vi "pH电极校准.vi"() -> ()   [LabVIEW 2016, in "国弘多参数.lvlib"]
uses:
  <vilib>/Analysis/NI_AALBase.lvlib
panel:
  out "变异系数":dbl
  out "standard deviation":dbl caption="标准差" format="%0.2f"
  out "mean":dbl caption="均值" format="%0.2f"
  out "当前检测值":dbl
  out "提示":string
  in  "第二点通过校正":bool
  in  "第一点通过校正":bool
  in  "第二点校正":bool
  in  "第一点校正":bool
  out "标液2":dbl
  out "标液1":dbl
  out "当前信号值":dbl
  out "偏移值补偿":dbl
  out "电极斜率":dbl
  out "电极零点":dbl
  # "酸碱度电极设定"
  # "mV"
  # "pH"
  # "%"
  # "mV"
  # "电极校正"
  # "标准液值:"
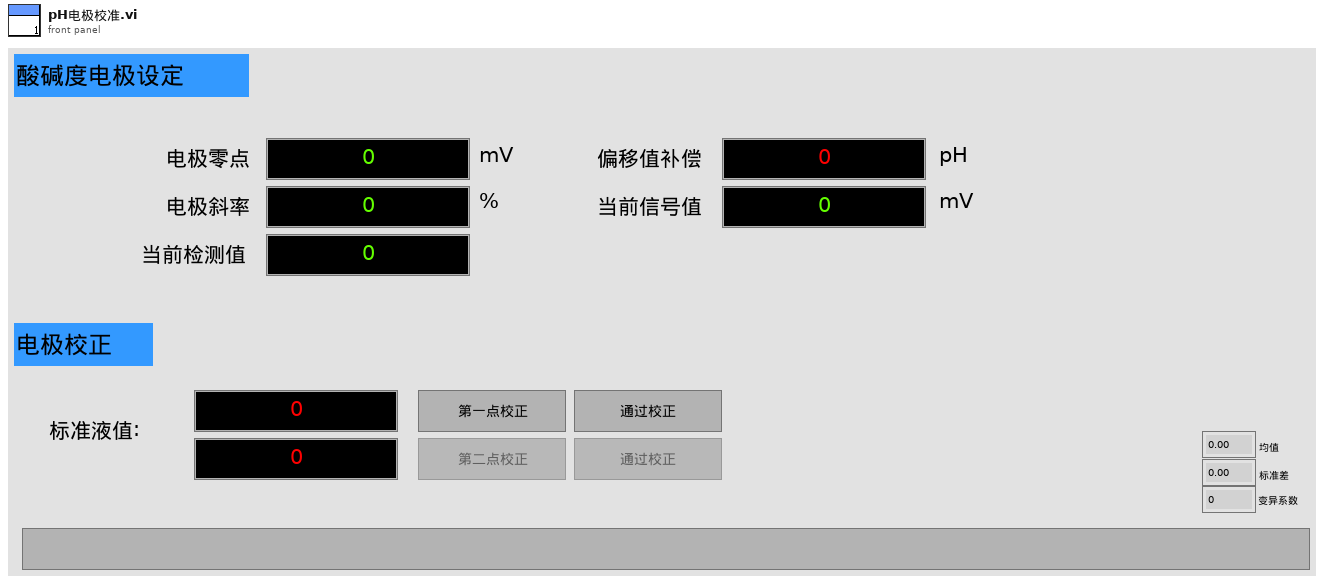
[diagram p1: front panel]
types:
  T1 = typedef "国弘多参数.lvlib/校准步骤.ctl" = enum16{"待机", "第一点校准启动", "第二点校准启动", "第一点校准写入", "第二点校准写入", "第一点校准失败", "第二点校准失败"}
  T2 = enum8{"Enabled", "Disabled", "Disabled and Grayed Out"}
  T3 = cluster{"电极状态标志":u16, "电极型号标志":u16, "酸碱度测量值":sgl, "温度测量值":sgl, "酸碱度信号值":sgl, "温度信号值":sgl, "酸碱度偏移修正值":sgl, "温度偏移修正值":sgl, "手动温度补偿值":sgl, "酸碱度电极零点":sgl, "酸碱度电极斜率":sgl, "第1点标准值记录":sgl, "第1点信号值记录":sgl, "第1点温度值记录":sgl, "第2点标准值记录":sgl, "第2点信号值记录":sgl, "第2点温度值记录":sgl, "命令滤波设定":u16, "温度模式":enum16{"ATC", "MTC"}, "生产批次":u16, "电极序号":u16, "串口地址":u16, "串口波特率":enum16{"9600", "19200", "115200"}, "串口校验位":enum16{"NONE", "ODD", "EVEN"}, "串口停止位":enum16{"1bit", "2bit"}, "第一点标准值":sgl, "第二点标准值":sgl}
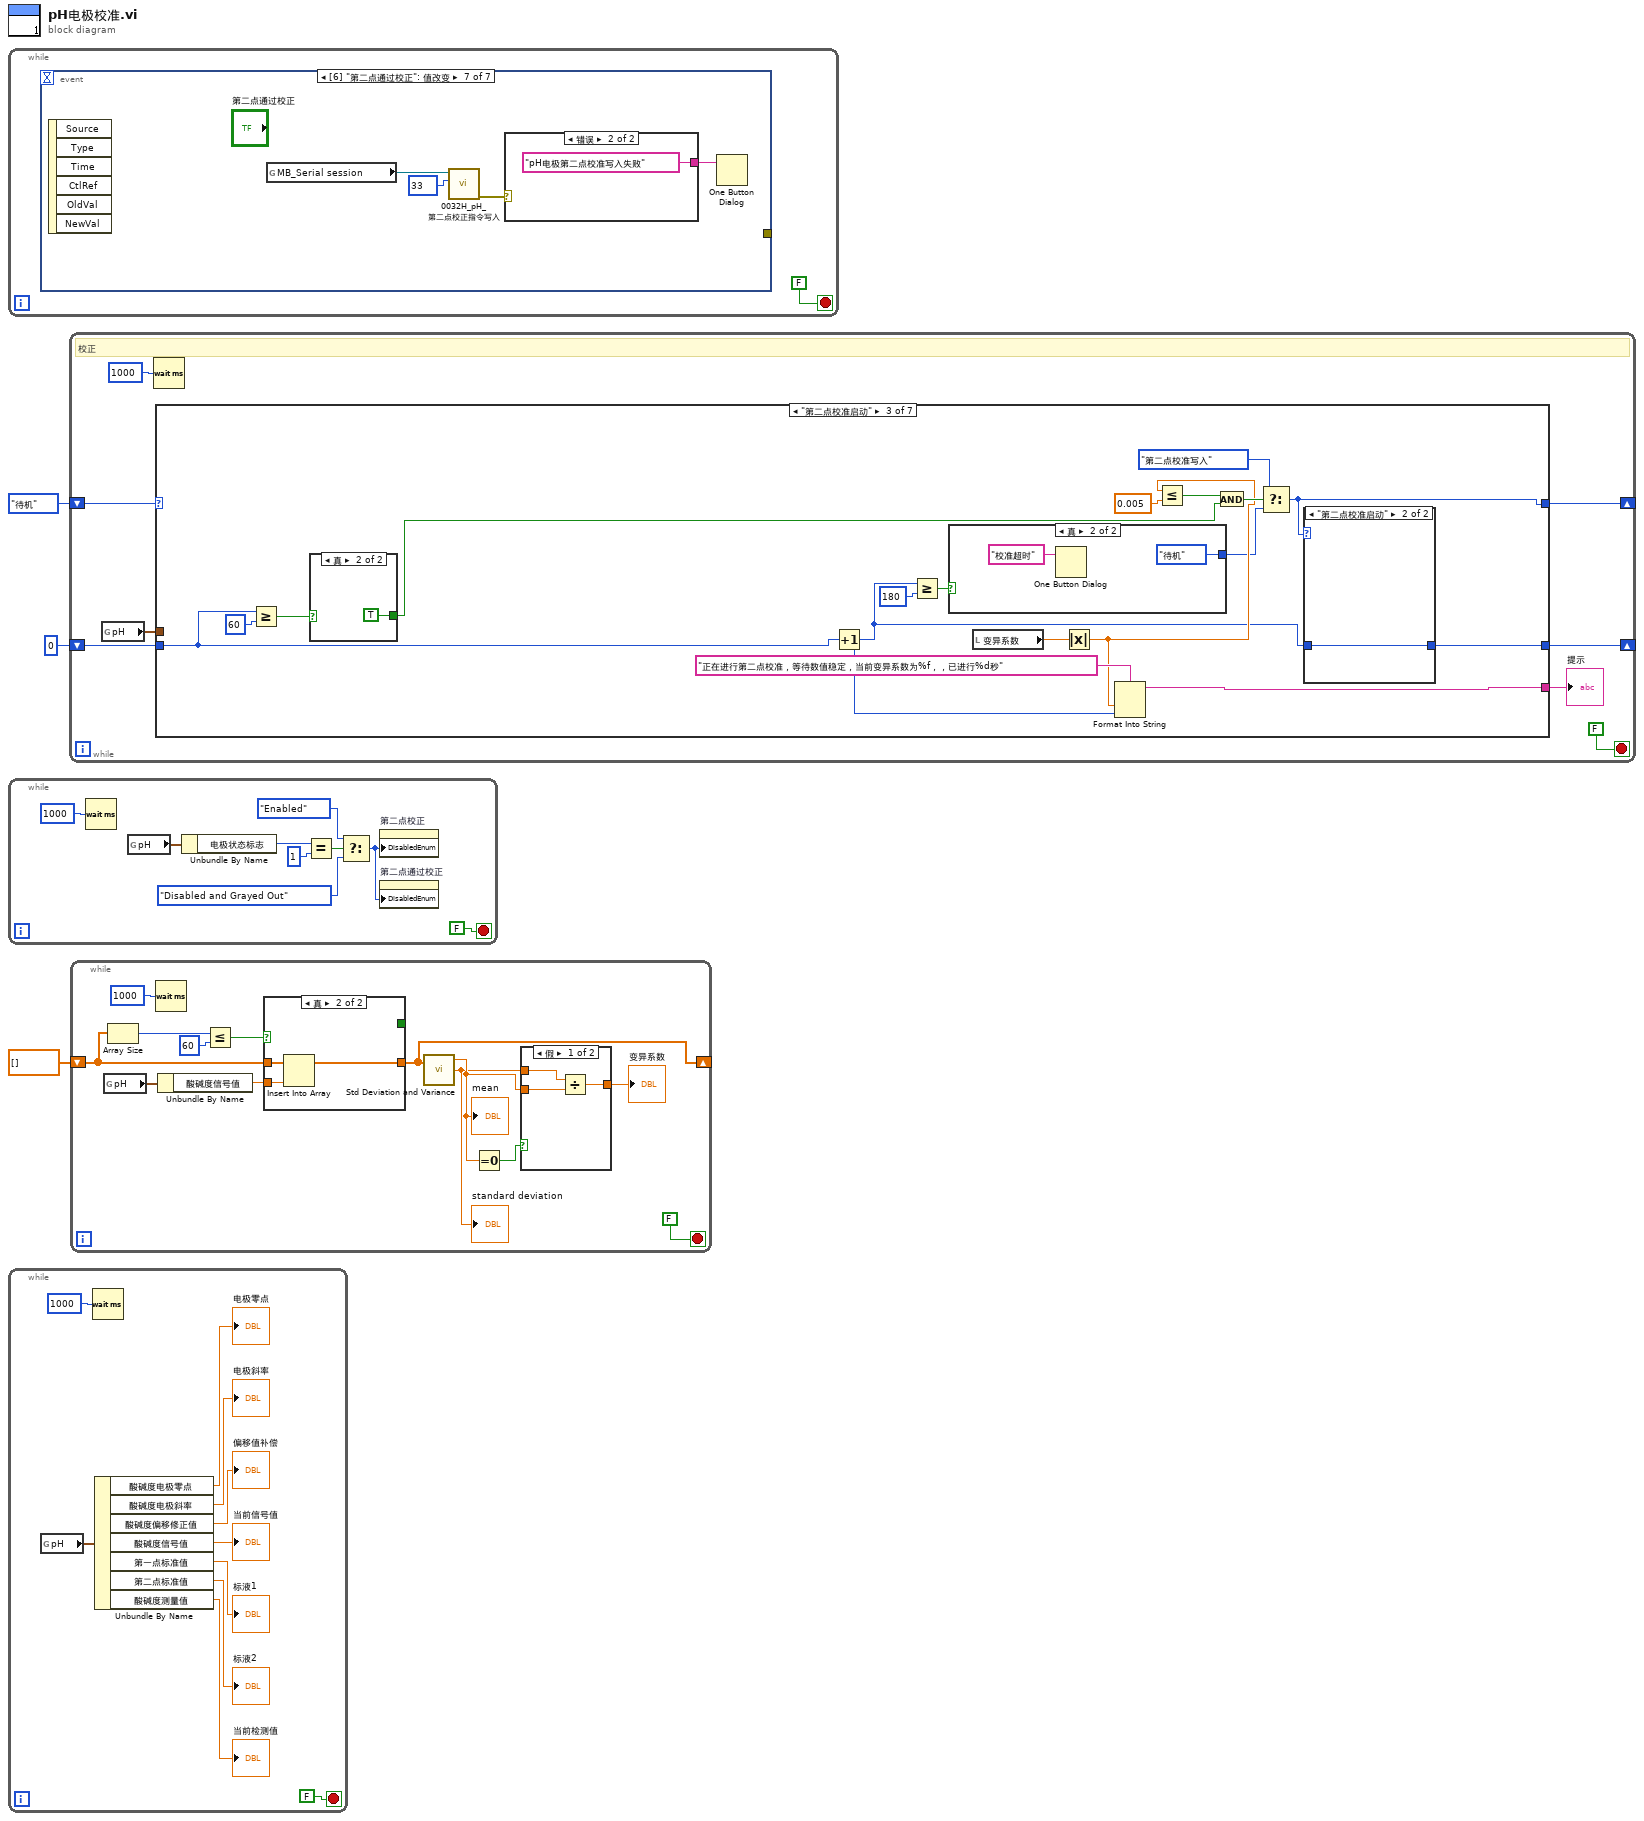
[diagram p0: block diagram]
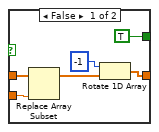
[diagram p3: hidden frame]
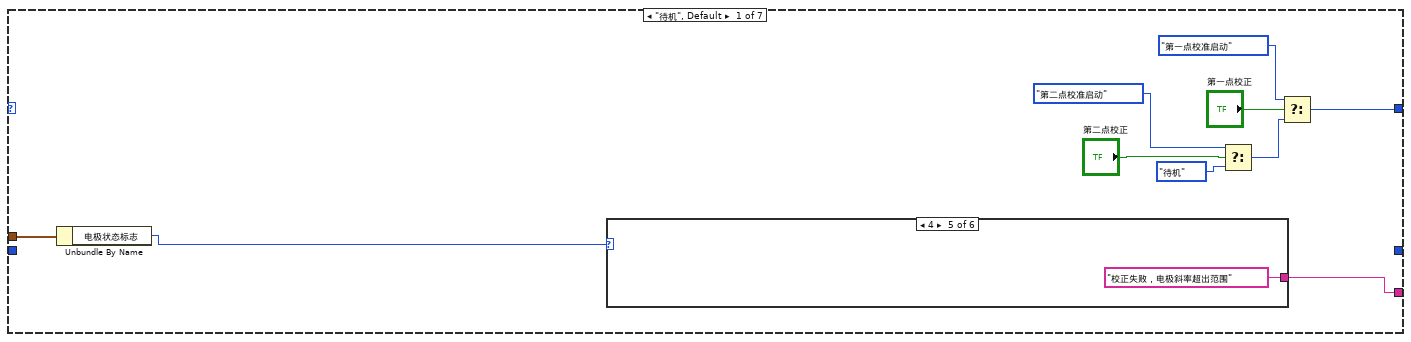
[diagram p4: hidden frame]
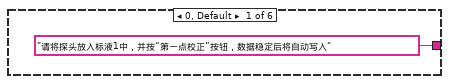
[diagram p5: hidden frame]
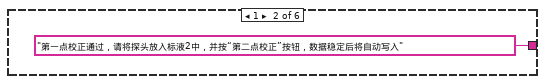
[diagram p6: hidden frame]
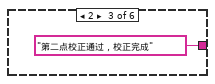
[diagram p7: hidden frame]
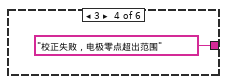
[diagram p8: hidden frame]
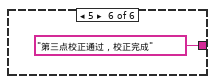
[diagram p9: hidden frame]
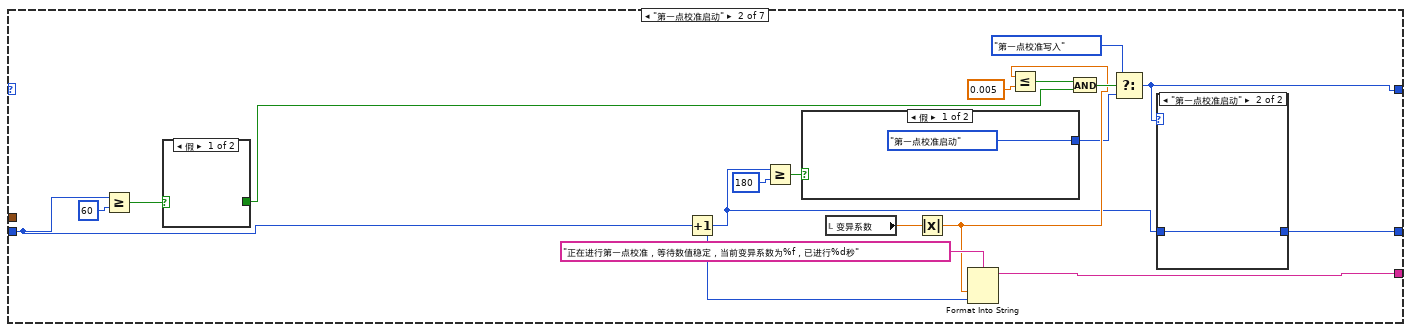
[diagram p10: hidden frame]
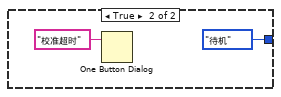
[diagram p12: hidden frame]
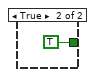
[diagram p13: hidden frame]
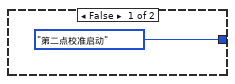
[diagram p15: hidden frame]
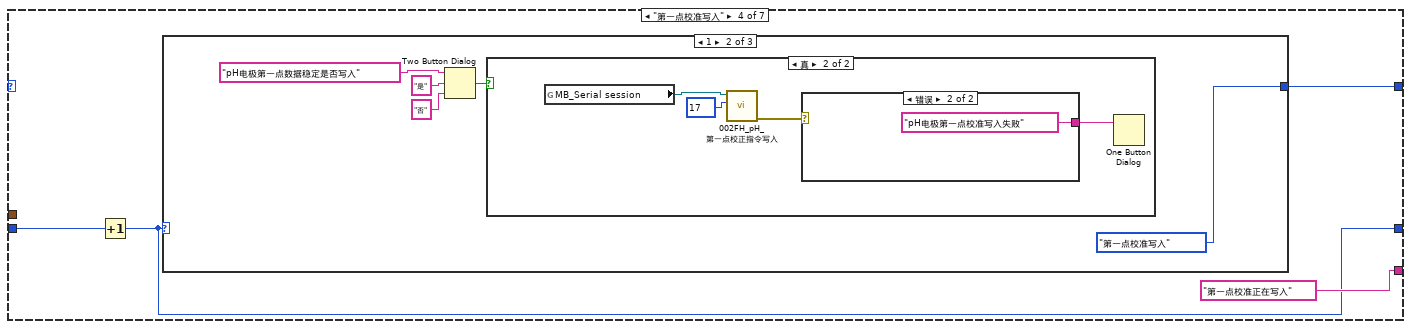
[diagram p17: hidden frame]
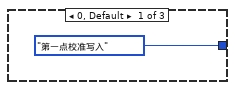
[diagram p18: hidden frame]
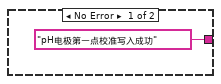
[diagram p20: hidden frame]
diagram:
  n1 = while {
    stop <- FALSE stop-if-true
    n2 = event shown="[6] \"第二点通过校正\": 值改变" {
      selector: _ -> [_ _ _ _ _ _ _]
      dyn-events: _ -> [_ _ _ _ _ _ _]
      timeout: _ -> [_ _ _ _ _ _ _]
      tunnel: [_ _ w9 w12 w15 _ _] -> _
      event Timeout {
        n3 = event-data() -> ()  [unwired: 1 in, 3 out]
      }
      event "标液1", "标液2", "偏移值补偿": Mouse Down {
        n4 = event-data() -> ("CtlRef"=w8:refnum<vi>)  [unwired: 1 in, 7 out]
        n5 = property class="DigNum (严格)"(reference=w8) -> (reference out=w5:refnum<vi>, "Value"=w6:dbl)  [unwired: 1 in, 1 out]
        n6 = call "数字键盘.vi"("OldNumber"=w6) -> ("NewNumber"=w7:sgl)
        n7 = property class="DigNum (严格)"(reference=w5, "Val(Sgnl)"=w7) -> ()  [unwired: 1 in, 2 out]
      }
      event "偏移值补偿": Value Change {
        n8 = event-data() -> ("NewVal"=w11:dbl)  [unwired: 1 in, 5 out]
        n9 = global read "过程全局变量.vi" "MB_Serial session"() -> (w10:refnum<class "MB_Master_Serial.lvclass">)
        n10 = call "000CH_pH_pH偏移修正值写入.vi"("数值"=w11, "MB_Serial session in"=w10) -> ("error out"=w9:errorcluster)  [unwired: 8 in, 1 out]
      }
      event "标液1": Value Change {
        n11 = event-data() -> ("NewVal"=w13:dbl)  [unwired: 1 in, 5 out]
        n12 = global read "过程全局变量.vi" "MB_Serial session"() -> (w14:refnum<class "MB_Master_Serial.lvclass">)
        n13 = call "0030H_pH_第一点标准值写入.vi"("数值"=w13, "MB_Serial session in"=w14) -> ("error out"=w12:errorcluster)  [unwired: 8 in, 1 out]
      }
      event "标液2": Value Change {
        n14 = event-data() -> ("NewVal"=w16:dbl)  [unwired: 1 in, 5 out]
        n15 = global read "过程全局变量.vi" "MB_Serial session"() -> (w17:refnum<class "MB_Master_Serial.lvclass">)
        n16 = call "0033H_pH_第二点标准值写入.vi"("数值"=w16, "MB_Serial session in"=w17) -> ("error out"=w15:errorcluster)  [unwired: 8 in, 1 out]
      }
      event "第一点通过校正": Value Change {
        n17 = event-data() -> ()  [unwired: 1 in, 6 out]
        n18 = global read "过程全局变量.vi" "MB_Serial session"() -> (w21:refnum<class "MB_Master_Serial.lvclass">)
        n19 = call "002FH_pH_第一点校正指令写入.vi"("数值"=u16 17, "MB_Serial session in"=w21) -> ("error out"=w18:errorcluster)  [unwired: 8 in, 1 out]
        n20 = case shown="错误" w18 {
          tunnel: ["pH电极第一点校准写入成功" ("消息") "pH电极第一点校准写入失败" ("消息")] -> w19
          frame No Error {
          }
          frame Error {
          }
        }
        n21 = One Button Dialog(message=w19) -> ()  [unwired: 1 in, 1 out]
      }
      event "第二点通过校正": Value Change {
        n22 = event-data() -> ()  [unwired: 1 in, 6 out]
        n23 = global read "过程全局变量.vi" "MB_Serial session"() -> (w27:refnum<class "MB_Master_Serial.lvclass">)
        n24 = call "0032H_pH_第二点校正指令写入.vi"("数值"=u16 33, "MB_Serial session in"=w27) -> ("error out"=w24:errorcluster)  [unwired: 8 in, 1 out]
        n25 = case shown="错误" w24 {
          tunnel: ["pH电极第二点校准写入成功" ("消息") "pH电极第二点校准写入失败" ("消息")] -> w25
          frame No Error {
          }
          frame Error {
          }
        }
        n26 = One Button Dialog(message=w25) -> ()  [unwired: 1 in, 1 out]
      }
    }
  }
  n27 = while {
    stop <- FALSE stop-if-true
    n28 = Wait (ms)(milliseconds to wait=u32 1000 ("等待时间（毫秒）")) -> ()  [unwired: 1 out]
    n29 = global read "过程全局变量.vi" "pH"() -> (w36:T3)
    n30 = Unbundle By Name(w36) -> ("电极状态标志"=w35:u16)
    n31 = Equal?(x=w35, y=u16 1) -> (x = y?=w30:bool)
    n32 = Select(t=T2."Enabled" ("禁用"), s=w30, f=T2."Disabled and Grayed Out" ("禁用")) -> (s? t:f=w31:T2)
    n33 = property on="第二点校正" class="Bool"("DisabledEnum"=w31) -> ()  [unwired: 2 in, 2 out]
    n34 = property on="第二点通过校正" class="Bool"("DisabledEnum"=w31) -> ()  [unwired: 2 in, 2 out]
  }
  n35 = while {
    stop <- FALSE stop-if-true
    n36 = global read "过程全局变量.vi" "pH"() -> (w46:T3)
    n37 = Wait (ms)(milliseconds to wait=u32 1000 ("等待时间（毫秒）")) -> ()  [unwired: 1 out]
    n38 = Unbundle By Name(w46) -> ("酸碱度电极零点"=→"电极零点":sgl, "酸碱度电极斜率"=→"电极斜率":sgl, "酸碱度偏移修正值"=→"偏移值补偿":sgl, "酸碱度信号值"=→"当前信号值":sgl, "第一点标准值"=→"标液1":sgl, "第二点标准值"=→"标液2":sgl, "酸碱度测量值"=→"当前检测值":sgl)
  }
  n39 = while "While循环" {
    shift-right: [w55] -> _
    shift-left: 校准步骤."待机" ("枚举") -> [w56]
    shift-right: [w50] -> _
    shift-left: 0 -> [w51]
    stop <- FALSE stop-if-true
    # "校正"
    n40 = global read "过程全局变量.vi" "pH"() -> (w49:T3)
    n41 = Wait (ms)(milliseconds to wait=u32 1000 ("等待时间（毫秒）")) -> ()  [unwired: 1 out]
    n42 = case shown="\"第二点校准启动\"" w56 {
      tunnel: [w64 w77 w100 w119 校准步骤."待机" ("枚举") 校准步骤."待机" ("枚举") 校准步骤."待机" ("枚举")] -> w55
      tunnel: [w62 w87 w105 "第一点校准正在写入" ("提示") "第二点校准正在写入" ("提示") "第一点校准失败" ("提示") "第二点校准失败" ("提示")] -> w53
      tunnel: w51 -> [_ w74 w97 w121 w137 w154 w159]
      tunnel: [_ w75 w98 w120 w136 w153 w158] -> w50
      tunnel: w49 -> [w57 _ _ _ _ _ _]
      frame "待机", Default {
        n43 = Unbundle By Name(w57) -> ("电极状态标志"=w63:u16)
        n44 = case shown="4" w63 {
          tunnel: ["请将探头放入标液1中，并按“第一点校正”按钮，数据稳定后将自动写入" ("提示") "第一点校正通过，请将探头放入标液2中，并按“第二点校正”按钮，数据稳定后将自动写入" ("提示") "第二点校正通过，校正完成" ("提示") "校正失败，电极零点超出范围" ("提示") "校正失败，电极斜率超出范围" ("提示") "第三点校正通过，校正完成" ("提示")] -> w62
          frame 0, Default {
          }
          frame 1 {
          }
          frame 2 {
          }
          frame 3 {
          }
          frame 4 {
          }
          frame 5 {
          }
        }
        n45 = Select(t=校准步骤."第二点校准启动" ("枚举"), s="第二点校正", f=校准步骤."待机" ("枚举")) -> (s? t:f=w58:T1)
        n46 = Select(t=校准步骤."第一点校准启动" ("枚举"), s="第一点校正", f=w58) -> (s? t:f=w64:T1)
      }
      frame "第一点校准启动" {
        n47 = Greater Or Equal?(x=w74, y=60) -> (x >= y?=w89:bool)
        n48 = case shown="假" w89 {
          tunnel: [_ TRUE] -> w84
          frame False {
          }
          frame True {
          }
        }
        n49 = Increment(x=w74) -> (x+1=w76:i32)
        n50 = Greater Or Equal?(x=w76, y=180) -> (x >= y?=w79:bool)
        n51 = case shown="假" w79 {
          tunnel: [校准步骤."第一点校准启动" ("枚举") 校准步骤."待机" ("枚举")] -> w78
          frame False {
          }
          frame True {
            n52 = One Button Dialog(message="校准超时" ("消息")) -> ()  [unwired: 1 in, 1 out]
          }
        }
        n53 = local read "变异系数"() -> (w73:dbl)
        n54 = Absolute Value(x=w73) -> (abs(x)=w81:dbl)
        n55 = Format Into String(format string="正在进行第一点校准，等待数值稳定，当前变异系数为%f，已进行%d秒" ("格式字符串"), w81, w76) -> (resulting string=w87:string)  [unwired: 2 in, 1 out]
        n56 = Less Or Equal?(x=w81, y=0.005) -> (x <= y?=w83:bool)
        n57 = And(x=w83, y=w84) -> (x .and. y?=w82:bool)
        n58 = Select(t=校准步骤."第一点校准写入" ("枚举"), s=w82, f=w78) -> (s? t:f=w77:T1)
        n59 = case shown="\"第一点校准启动\"" w77 {
          tunnel: w76 -> [_ w91]
          tunnel: [_ w91] -> w75
          frame "待机", Default {
          }
          frame "第一点校准启动" {
          }
        }
      }
      frame "第二点校准启动" {
        n60 = Greater Or Equal?(x=w97, y=60) -> (x >= y?=w112:bool)
        n61 = case shown="真" w112 {
          tunnel: [_ TRUE] -> w108
          frame False {
          }
          frame True {
          }
        }
        n62 = Increment(x=w97) -> (x+1=w99:i32)
        n63 = Greater Or Equal?(x=w99, y=180) -> (x >= y?=w102:bool)
        n64 = case shown="真" w102 {
          tunnel: [校准步骤."第二点校准启动" ("枚举") 校准步骤."待机" ("枚举")] -> w101
          frame False {
          }
          frame True {
            n65 = One Button Dialog(message="校准超时" ("消息")) -> ()  [unwired: 1 in, 1 out]
          }
        }
        n66 = local read "变异系数"() -> (w96:dbl)
        n67 = Absolute Value(x=w96) -> (abs(x)=w104:dbl)
        n68 = Format Into String(format string="正在进行第二点校准，等待数值稳定，当前变异系数为%f，，已进行%d秒" ("格式字符串"), w104, w99) -> (resulting string=w105:string)  [unwired: 2 in, 1 out]
        n69 = Less Or Equal?(x=w104, y=0.005) -> (x <= y?=w107:bool)
        n70 = And(x=w107, y=w108) -> (x .and. y?=w106:bool)
        n71 = Select(t=校准步骤."第二点校准写入" ("枚举"), s=w106, f=w101) -> (s? t:f=w100:T1)
        n72 = case shown="\"第二点校准启动\"" w100 {
          tunnel: w99 -> [_ w114]
          tunnel: [_ w114] -> w98
          frame "待机", Default {
          }
          frame "第二点校准启动" {
          }
        }
      }
      frame "第一点校准写入" {
        n73 = Increment(x=w121) -> (x+1=w120:i32)
        n74 = case shown="1" w120 {
          tunnel: [校准步骤."第一点校准写入" ("枚举") 校准步骤."第一点校准写入" ("枚举") 校准步骤."待机" ("枚举")] -> w119
          frame 0, Default {
          }
          frame 1 {
            n75 = Two Button Dialog(message="pH电极第一点数据稳定是否写入" ("消息"), 1:"否" ("F按钮名称（“取消”）"), 2:"是" ("T按钮名称（“确定”）")) -> (T button?=w124:bool)
            n76 = case shown="真" w124 {
              frame False {
              }
              frame True {
                n77 = global read "过程全局变量.vi" "MB_Serial session"() -> (w131:refnum<class "MB_Master_Serial.lvclass">)
                n78 = call "002FH_pH_第一点校正指令写入.vi"("数值"=u16 17, "MB_Serial session in"=w131) -> ("error out"=w129:errorcluster)  [unwired: 8 in, 1 out]
                n79 = case shown="错误" w129 {
                  tunnel: ["pH电极第一点校准写入成功" ("消息") "pH电极第一点校准写入失败" ("消息")] -> w130
                  frame No Error {
                  }
                  frame Error {
                  }
                }
                n80 = One Button Dialog(message=w130) -> ()  [unwired: 1 in, 1 out]
              }
            }
          }
          frame 2 {
          }
        }
      }
      frame "第二点校准写入" {
        n81 = Increment(x=w137) -> (x+1=w136:i32)
        n82 = case shown="1" w136 {
          tunnel: [校准步骤."第二点校准写入" ("枚举") 校准步骤."第二点校准写入" ("枚举") 校准步骤."待机" ("枚举")] -> _
          frame 0, Default {
          }
          frame 1 {
            n83 = Two Button Dialog(message="pH电极第二点数据稳定是否写入" ("消息"), 1:"否" ("F按钮名称（“取消”）"), 2:"是" ("T按钮名称（“确定”）")) -> (T button?=w141:bool)
            n84 = case shown="真" w141 {
              frame False {
              }
              frame True {
                n85 = global read "过程全局变量.vi" "MB_Serial session"() -> (w149:refnum<class "MB_Master_Serial.lvclass">)
                n86 = call "0032H_pH_第二点校正指令写入.vi"("数值"=u16 33, "MB_Serial session in"=w149) -> ("error out"=w147:errorcluster)  [unwired: 8 in, 1 out]
                n87 = case shown="错误" w147 {
                  tunnel: ["pH电极第二点校准写入成功" ("消息") "pH电极第二点校准写入失败" ("消息")] -> w146
                  frame No Error {
                  }
                  frame Error {
                  }
                }
                n88 = One Button Dialog(message=w146) -> ()  [unwired: 1 in, 1 out]
              }
            }
          }
          frame 2 {
          }
        }
      }
      frame "第一点校准失败" {
        n89 = Two Button Dialog(message="第一点校准失败是否重新校准" ("消息")) -> ()  [unwired: 2 in, 1 out]
        n90 = Increment(x=w154) -> (x+1=w153:i32)
      }
      frame "第二点校准失败" {
        n91 = Increment(x=w159) -> (x+1=w158:i32)
      }
    }
    "提示" <- w53
  }
  n92 = while {
    shift-right: [w167] -> _
    shift-left: sgl[] [] -> [w170]
    stop <- FALSE stop-if-true
    n93 = global read "过程全局变量.vi" "pH"() -> (w162:T3)
    n94 = Array Size(array=w170) -> (size(s)=w172:i32)
    n95 = Wait (ms)(milliseconds to wait=u32 1000 ("等待时间（毫秒）")) -> ()  [unwired: 1 out]
    n96 = Unbundle By Name(w162) -> ("酸碱度信号值"=w169:sgl)
    n97 = Less Or Equal?(x=w172, y=60) -> (x <= y?=w171:bool)
    n98 = case shown="真" w171 {
      tunnel: w170 -> [w183 w186]
      tunnel: w169 -> [w181 w185]
      tunnel: [w179 w184] -> w167
      tunnel: [TRUE _] -> _
      frame False {
        n99 = Replace Array Subset(array=w183, new element=w181) -> (w182:sgl[])  [unwired: 1 in]
        n100 = Rotate 1D Array(1:w182, 2:-1 ("n")) -> (0:w179:sgl[])
      }
      frame True {
        n101 = Insert Into Array(array=w186, new element=w185) -> (w184:sgl[])  [unwired: 1 in]
      }
    }
    n102 = call <vilib>:"Std Deviation and Variance.vi"("X"=w167) -> ("mean"=w166:dbl, "standard deviation"=w165:dbl)  [unwired: 1 in, 1 out]
    "mean" <- w166
    "standard deviation" <- w165
    n103 = Equal To 0?(x=w166) -> (x = 0?=w168:bool)
    n104 = case shown="假" w168 {
      tunnel: w165 -> [w177 _]
      tunnel: [w176 _] -> w164
      tunnel: w166 -> [w175 _]
      frame False {
        n105 = Divide(x=w177, y=w175) -> (x/y=w176:dbl)
      }
      frame True {
      }
    }
    "变异系数" <- w164
  }
